vi "Shift X kinetics.vi"(6 "shift":dbl=0.5 format="%#_13g", 8 "error in (no error)":errorcluster, 9 "#kinetics":i32=2 min=2 step=1, 10 "Combo Box":string(combo)="Kinetics", 11 "Control-Client in":refnum<class "Control-Client.lvclass">) -> (0 "error out":errorcluster, 3 "Control-Client out":refnum<class "Control-Client.lvclass">)   [LabVIEW 2018, in "Control-Client.lvclass"]
uses:
  Control-Client.lvclass
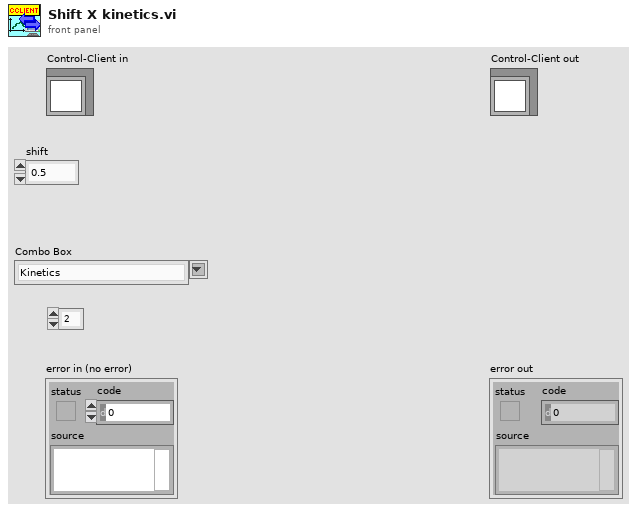
[diagram p1: front panel]
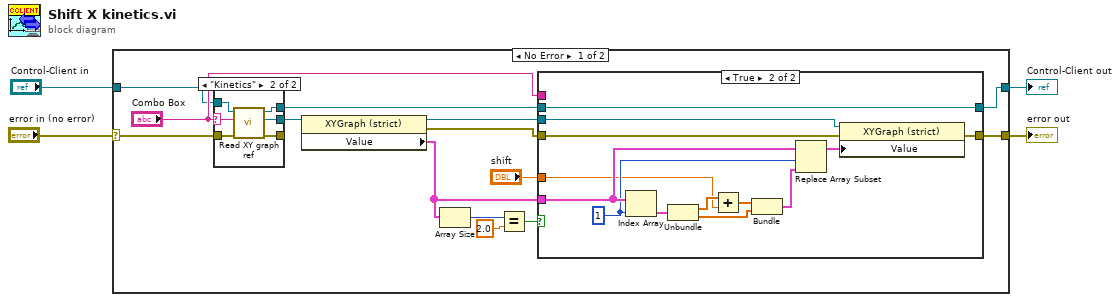
[diagram p0: block diagram]
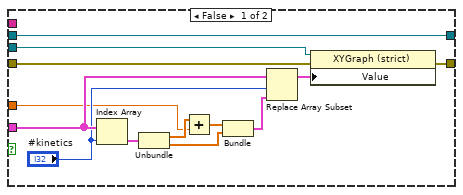
[diagram p2: hidden frame]
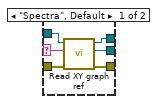
[diagram p3: hidden frame]
diagram:
  n1 = case shown="No Error" "error in (no error)" {
    selector: "error in (no error)" -> [w6 w58]
    tunnel: "Control-Client in" -> [w7 w57]
    tunnel: [w14 w58] -> w3
    tunnel: [w13 w57] -> w2
    frame No Error {
      n2 = case shown="\"Kinetics\"" "Combo Box" {
        selector: "Combo Box" -> [w50 w53]
        tunnel: [w48 w56] -> w17
        tunnel: [w47 w55] -> _
        tunnel: w7 -> [w49 w54]
        tunnel: [w46 w52] -> w18
        tunnel: w6 -> [w45 w51]
        frame "Spectra", Default {
          n3 = call "Read XY graph ref.vi"("error in (no error)"=w45, "Combo Box"=w50, "Control-Client in"=w49) -> ("error out"=w47:errorcluster, "XY graph ref"=w48:refnum<vi>, "Control-Client out"=w46:refnum<class "Control-Client.lvclass">)  [unwired: 6 in]
        }
        frame "Kinetics" {
          n4 = call "Read XY graph ref.vi"("error in (no error)"=w51, "Combo Box"=w53, "Control-Client in"=w54) -> ("error out"=w55:errorcluster, "XY graph ref"=w56:refnum<vi>, "Control-Client out"=w52:refnum<class "Control-Client.lvclass">)  [unwired: 6 in]
        }
      }
      n5 = property class="XYGraph (strict)"(reference=w17) -> (reference out=w16:refnum<vi>, error out=w15:errorcluster, "Value"=w11:cluster{"Y":dbl[], "Y":dbl[]}[])  [unwired: 1 in]
      n6 = Array Size(array=w11) -> (size(s)=w10:i32)
      n7 = Equal?(x=w10, y=2.0) -> (x = y?=w9:bool)
      n8 = case shown="True" w9 {
        tunnel: w18 -> [w25 w39]
        tunnel: w16 -> [w31 w44]
        tunnel: w11 -> [w28 w41]
        tunnel: w15 -> [w30 w43]
        tunnel: [w24 w38] -> w14
        tunnel: [w25 w39] -> w13
        tunnel: "Combo Box" -> [_ _]
        tunnel: "shift" -> [w19 w32]
        frame False {
          n9 = Index Array(array=w28, index="#kinetics") -> (element=w29:cluster{"Y":dbl[], "Y":dbl[]})
          n10 = Unbundle(w29) -> ("Y"=w23:dbl[], "Y"=w22:dbl[])
          n11 = Add(x=w23, y=w19) -> (x+y=w21:dbl[])
          n12 = Bundle(w21, "Y"=w22) -> (w20:cluster{dbl[], "Y":dbl[]})  [unwired: 1 in]
          n13 = Replace Array Subset(array=w28, new element=w20, index="#kinetics") -> (w27:cluster{"Y":dbl[], "Y":dbl[]}[])
          n14 = property class="XYGraph (strict)"(reference=w31, error in=w30, "Value"=w27) -> (error out=w24:errorcluster)  [unwired: 1 out]
        }
        frame True {
          w33 = 1 ("index")
          n15 = Index Array(array=w41, index=w33) -> (element=w42:cluster{"Y":dbl[], "Y":dbl[]})
          n16 = Unbundle(w42) -> ("Y"=w37:dbl[], "Y"=w36:dbl[])
          n17 = Add(x=w37, y=w32) -> (x+y=w35:dbl[])
          n18 = Bundle(w35, "Y"=w36) -> (w34:cluster{dbl[], "Y":dbl[]})  [unwired: 1 in]
          n19 = Replace Array Subset(array=w41, new element=w34, index=w33) -> (w40:cluster{"Y":dbl[], "Y":dbl[]}[])
          n20 = property class="XYGraph (strict)"(reference=w44, error in=w43, "Value"=w40) -> (error out=w38:errorcluster)  [unwired: 1 out]
        }
      }
    }
    frame Error {
    }
  }
  "error out" <- w3
  "Control-Client out" <- w2
